vi "VSI Write Bits.vi"(7 "pWriteBitStr":string, 8 "error in (no error)":errorcluster, 9 "SPIIndex":i32, 10 "DevIndex":i32, 11 "DevType":i32) -> (0 "error out":errorcluster, 3 "function return":i32)   [LabVIEW 2012, in "ControlSPI.lvlib"]
doc: "int WINAPI VSI_WriteBits(int DevType,int DevIndex,int SPIIndex,unsigned char *pWriteBitStr);"
uses:
  ControlSPI.lvlib
  Ginkgo_Driver.dll
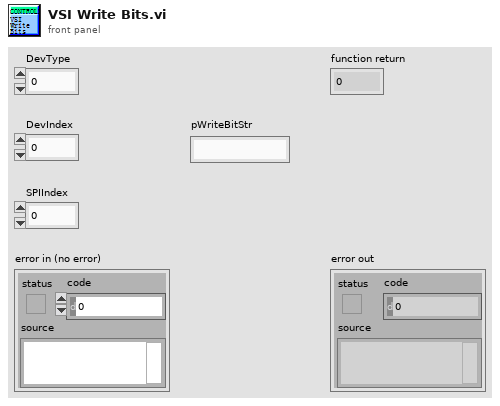
[diagram p1: front panel]
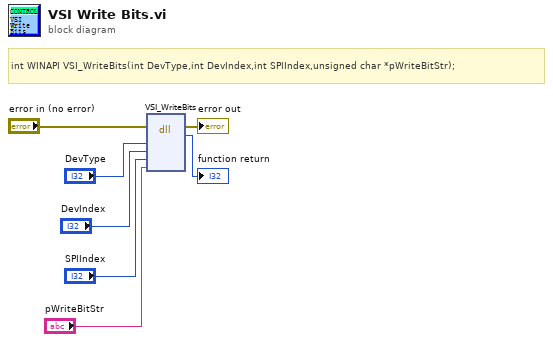
[diagram p0: block diagram]
diagram:
  # "int WINAPI VSI_WriteBits(int DevType,int DevIndex,int SPIIndex,unsigned char *pWriteBitStr);"
  n1 = dll-call lib="E:/Project/vt_ginkgo/truck/Ginkgo Driver/vs2010/Ginkgo_USB-I2C_API_v2.0.3.0/lib/labview_32bit/ControlSPI/Ginkgo_Driver.*" fn="VSI_WriteBits"(error in="error in (no error)", "DevType"="DevType", "DevIndex"="DevIndex", "SPIIndex"="SPIIndex", "pWriteBitStr"="pWriteBitStr") -> (error out=→"error out":errorcluster, →"function return":i32)  [unwired: 6 in, 1 out]
